vi "Write Identifier.vi"(0 "Session Handle in":T1, 5 "identifier":u16, 11 "error in (no error)":errorcluster) -> (4 "Session Handle out":T1, 15 "error out":errorcluster)   [LabVIEW 2015, in "PAS.lvclass"]
uses:
  PAS.lvclass
  Typedefs/Session Handle.ctl
  PAS.lvclass/PAS.ctl
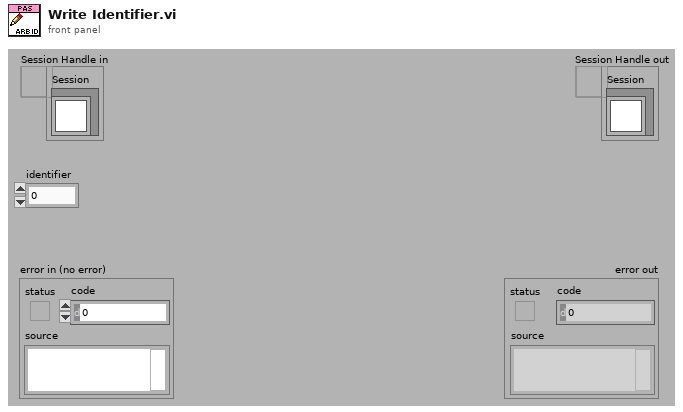
[diagram p1: front panel]
types:
  T1 = typedef "PAS.lvclass/Session Handle.ctl" = refnum<data-value>
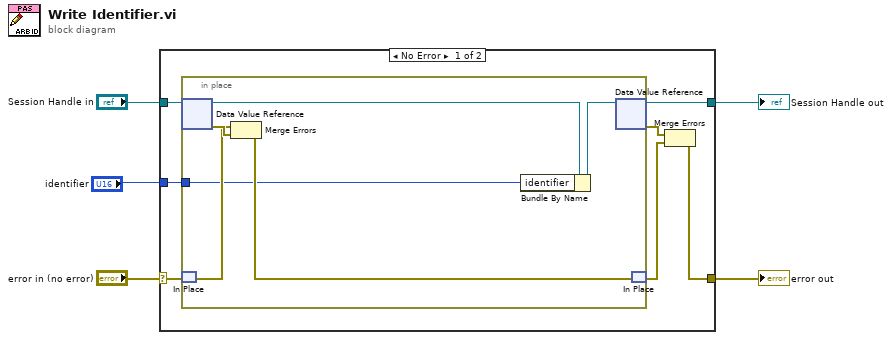
[diagram p0: block diagram]
diagram:
  n1 = case shown="No Error" "error in (no error)" {
    selector: "error in (no error)" -> [w7 w19]
    tunnel: "Session Handle in" -> [w12 w20]
    tunnel: [w11 w20] -> w4
    tunnel: [w8 w19] -> w3
    tunnel: "identifier" -> [w6 _]
    frame No Error {
      n2 = in-place {
        in-place-border: w6 -> [w13]
        n3 = in-place-dvr #1(w12) -> (w15:refnum<class "PAS.lvclass">, w17:errorcluster)
        n4 = in-place-match #2(w7) -> (w16:errorcluster)
        n5 = Merge Errors(w16, w17) -> (w18:errorcluster)
        n6 = Bundle By Name(cluster=w15, "identifier"=w13) -> (w14:refnum<class "PAS.lvclass">)
        n7 = in-place-dvr #1(w14) -> (w11:T1, w9:errorcluster)
        n8 = in-place-match #2(w18) -> (w10:errorcluster)
      }
      n9 = Merge Errors(w9, w10) -> (w8:errorcluster)
    }
    frame Error {
    }
  }
  "Session Handle out" <- w4
  "error out" <- w3
